vi "List Available Cylinders for Knock Sensor.vi"(8 "error in (no error)":errorcluster, 10 "Timing measurement":string, 11 "Item Ref in":T1 format="%.0x") -> (0 "error out":errorcluster, 2 "cylinders available":string[](array[string]), 3 "Item Ref out":T1 format="%.0x")   [LabVIEW 2019, in "Engine Simulation Toolkit System Explorer.lvlib"]
uses:
  Engine Simulation Toolkit System Explorer.lvlib
  <vilib>/NI VeriStand/Custom Device API/Custom Device Item Ref.ctl
  Shared/Properties.vi
  Shared/Engine Simulation Toolkit Shared.lvlib
  <vilib>/NI VeriStand/Custom Device API/Custom Device API.lvlib
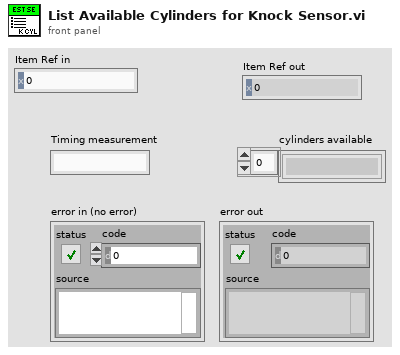
[diagram p1: front panel]
types:
  T1 = typedef "Custom Device API.lvlib/Custom Device Item Ref.ctl" = u64
  T2 = typedef "Custom Device API.lvlib/Custom Device Item Info.ctl" = cluster{"Name":string, "Is Channel":bool, "GUID":string, "Is Waveform":bool}
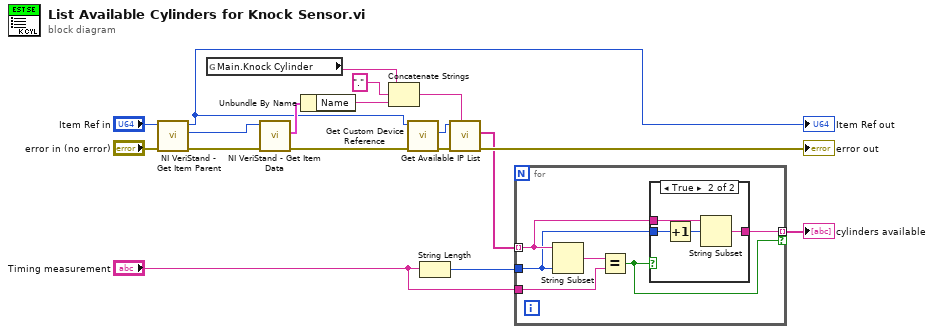
[diagram p0: block diagram]
diagram:
  n1 = call <vilib>:"NI VeriStand - Get Item Parent.vi"("error in (no error)"="error in (no error)", "Item Ref in"="Item Ref in") -> ("error out"=w7:errorcluster, "Parent Ref"=w8:T1, "Item Ref out"=w1:T1)  [unwired: 6 in, 1 out]
  "Item Ref out" <- w1
  n2 = global read "Properties.vi" "Main.Knock Cylinder"() -> (w4:string)
  n3 = call <vilib>:"NI VeriStand - Get Item Data.vi"("error in (no error)"=w7, "Item Ref in"=w8) -> ("error out"=w11:errorcluster, "Item Info"=w6:T2)  [unwired: 6 in, 2 out]
  n4 = Unbundle By Name(w6) -> ("Name"=w5:string)
  n5 = Concatenate Strings(w4, "." ("string"), w5) -> (w2:string)
  n6 = call "Get Custom Device Reference.vi"("error in (no error)"=w11, "Item Ref in"=w1) -> ("error out"=w12:errorcluster, "Custom Device Ref"=w13:T1)  [unwired: 7 in, 1 out]
  n7 = String Length(string="Timing measurement") -> (length=w16:i32)
  n8 = call "Get Available IP List.vi"("ip list property name"=w2, "error in (no error)"=w12, "Item Ref in"=w13) -> ("error out"=→"error out":errorcluster, "ips available"=w17:string[])  [unwired: 6 in, 1 out]
  n9 = for {
    tunnel: w17 -> [w22] mode=indexing
    tunnel: w16 -> [w21]
    tunnel: "Timing measurement" -> [w23]
    tunnel: [w20] -> w14 mode=indexing if=w19
    n10 = String Subset(string=w22, length (rest)=w21) -> (substring=w24:string)  [unwired: 1 in]
    n11 = Equal?(x=w24, y=w23) -> (x = y?=w19:bool)
    n12 = case shown="True" w19 {
      tunnel: w22 -> [_ w28]
      tunnel: w21 -> [_ w26]
      tunnel: [_ w27] -> w20
      frame False {
      }
      frame True {
        n13 = Increment(x=w26) -> (x+1=w25:i32)
        n14 = String Subset(string=w28, offset (0)=w25) -> (substring=w27:string)  [unwired: 1 in]
      }
    }
  }
  "cylinders available" <- w14
